vi "formatOutputwithTemperature.vi"(8 "error in (no error)":errorcluster, 11 "Electrometer in":refnum<class "Electrometer.lvclass">) -> (0 "error out":errorcluster, 3 "Electrometer out":refnum<class "Electrometer.lvclass">)   [LabVIEW 2016, in "Electrometer.lvclass"]
uses:
  Electrometer.lvclass
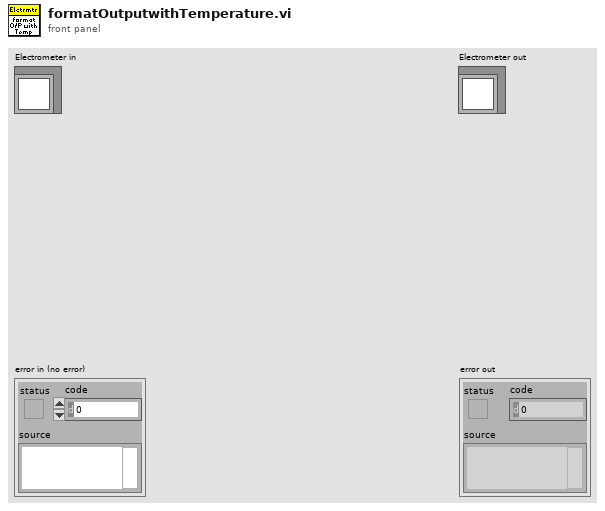
[diagram p1: front panel]
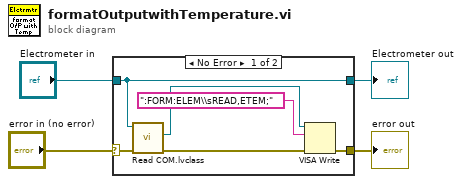
[diagram p0: block diagram]
diagram:
  n1 = case shown="No Error" "error in (no error)" {
    selector: "error in (no error)" -> [w7 w12]
    tunnel: [w6 w12] -> w3
    tunnel: [w9 w11] -> w1
    tunnel: "Electrometer in" -> [w9 w11]
    frame No Error {
      n2 = call "Read COM.lvclass.vi"("error in (no error)"=w7, "Electrometer in"=w9) -> ("error out"=w8:errorcluster, "VISA"=w5:refnum<visa-resource-name>)  [unwired: 7 in, 1 out]
      n3 = VISA Write(VISA resource name=w5, write buffer=":FORM:ELEM\\sREAD,ETEM;", error in (no error)=w8) -> (error out=w6:errorcluster)  [unwired: 2 out]
    }
    frame Error {
    }
  }
  "error out" <- w3
  "Electrometer out" <- w1
